vi "AD模拟量输入.vi"() -> ()   [LabVIEW 2010]
panel:
  in  "btn_反选":bool
  in  "btn_全选":bool
  in  "AD_16_5":sgl format="%.2f"
  in  "AD_16_4":sgl format="%.2f"
  in  "AD_16_3":sgl format="%.2f"
  in  "AD_16_2":sgl format="%.2f"
  in  "AD_16_1":sgl format="%.2f"
  in  "AD_15_5":sgl format="%.2f"
  in  "AD_15_4":sgl format="%.2f"
  in  "AD_15_3":sgl format="%.2f"
  in  "AD_15_2":sgl format="%.2f"
  in  "单选_AD_16":bool
  in  "单选_AD_15":bool
  in  "AD_15_1":sgl format="%.2f"
  in  "AD_14_5":sgl format="%.2f"
  in  "AD_14_4":sgl format="%.2f"
  in  "AD_14_3":sgl format="%.2f"
  in  "AD_14_2":sgl format="%.2f"
  in  "AD_14_1":sgl format="%.2f"
  in  "AD_13_5":sgl format="%.2f"
  in  "AD_13_4":sgl format="%.2f"
  in  "AD_13_3":sgl format="%.2f"
  in  "AD_13_2":sgl format="%.2f"
  in  "单选_AD_14":bool
  in  "单选_AD_13":bool
  in  "AD_13_1":sgl format="%.2f"
  in  "AD_12_5":sgl format="%.2f"
  in  "AD_12_4":sgl format="%.2f"
  in  "AD_12_3":sgl format="%.2f"
  in  "AD_12_2":sgl format="%.2f"
  in  "AD_12_1":sgl format="%.2f"
  in  "AD_11_5":sgl format="%.2f"
  in  "AD_11_4":sgl format="%.2f"
  in  "AD_11_3":sgl format="%.2f"
  in  "AD_11_2":sgl format="%.2f"
  in  "单选_AD_12":bool
  in  "单选_AD_11":bool
  in  "AD_11_1":sgl format="%.2f"
  in  "AD_10_5":sgl format="%.2f"
  in  "AD_10_4":sgl format="%.2f"
  in  "AD_10_3":sgl format="%.2f"
  in  "AD_10_2":sgl format="%.2f"
  in  "AD_10_1":sgl format="%.2f"
  in  "AD_9_5":sgl format="%.2f"
  in  "AD_9_4":sgl format="%.2f"
  in  "AD_9_3":sgl format="%.2f"
  in  "AD_9_2":sgl format="%.2f"
  in  "单选_AD_10":bool
  in  "单选_AD_9":bool
  in  "AD_9_1":sgl format="%.2f"
  in  "AD_8_5":sgl format="%.2f"
  in  "AD_8_4":sgl format="%.2f"
  in  "AD_8_3":sgl format="%.2f"
  in  "AD_8_2":sgl format="%.2f"
  in  "AD_8_1":sgl format="%.2f"
  in  "AD_7_5":sgl format="%.2f"
  in  "AD_7_4":sgl format="%.2f"
  in  "AD_7_3":sgl format="%.2f"
  in  "AD_7_2":sgl format="%.2f"
  in  "单选_AD_8":bool
  in  "单选_AD_7":bool
  in  "AD_7_1":sgl format="%.2f"
  in  "AD_6_5":sgl format="%.2f"
  in  "AD_6_4":sgl format="%.2f"
  in  "AD_6_3":sgl format="%.2f"
  in  "AD_6_2":sgl format="%.2f"
  in  "AD_6_1":sgl format="%.2f"
  in  "AD_5_5":sgl format="%.2f"
  in  "AD_5_4":sgl format="%.2f"
  in  "AD_5_3":sgl format="%.2f"
  in  "AD_5_2":sgl format="%.2f"
  in  "单选_AD_6":bool
  in  "单选_AD_5":bool
  in  "AD_5_1":sgl format="%.2f"
  in  "AD_4_5":sgl format="%.2f"
  in  "AD_4_4":sgl format="%.2f"
  in  "AD_4_3":sgl format="%.2f"
  in  "AD_4_2":sgl format="%.2f"
  in  "AD_4_1":sgl format="%.2f"
  in  "AD_3_5":sgl format="%.2f"
  in  "AD_3_4":sgl format="%.2f"
  in  "AD_3_3":sgl format="%.2f"
  in  "AD_3_2":sgl format="%.2f"
  in  "单选_AD_4":bool
  in  "单选_AD_3":bool
  in  "AD_3_1":sgl format="%.2f"
  in  "AD_2_5":sgl format="%.2f"
  in  "AD_2_4":sgl format="%.2f"
  in  "AD_2_3":sgl format="%.2f"
  in  "AD_2_2":sgl format="%.2f"
  in  "AD_2_1":sgl format="%.2f"
  in  "AD_1_5":sgl format="%.2f"
  in  "AD_1_4":sgl format="%.2f"
  in  "AD_1_3":sgl format="%.2f"
  in  "AD_1_2":sgl format="%.2f"
  in  "单选_AD_2":bool
  in  "单选_AD_1":bool
  in  "AD_1_1":sgl format="%.2f"
  in  "btn_取消":bool
  in  "btn_开始测试":bool
  # "第1路"
  # "输入值："
  # "输入值："
  # "第2路"
  # "第3路"
  # "输入值："
  # "输入值："
  # "第4路"
  # "第5路"
  # "输入值："
  # "输入值："
  # "第6路"
  # "第7路"
  # "输入值："
  # "输入值："
  # "第8路"
  # "第9路"
  # "输入值："
  # "输入值："
  # "第10路"
  # "第11路"
  # "输入值："
  # "输入值："
  # "第12路"
  # "第13路"
  # "输入值："
  # "输入值："
  # "第14路"
  # "第15路"
  # "输入值："
  # "输入值："
  # "第16路"
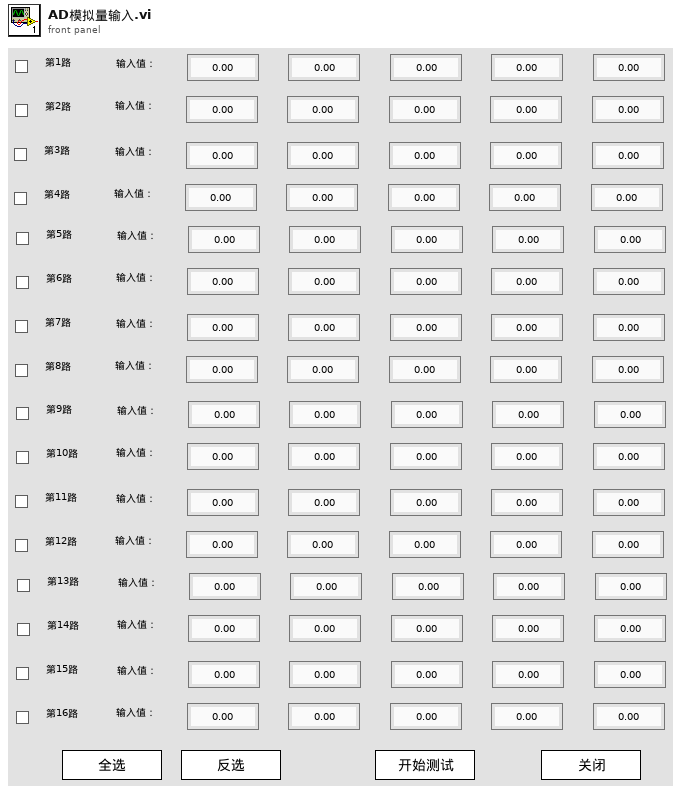
[diagram p1: front panel]
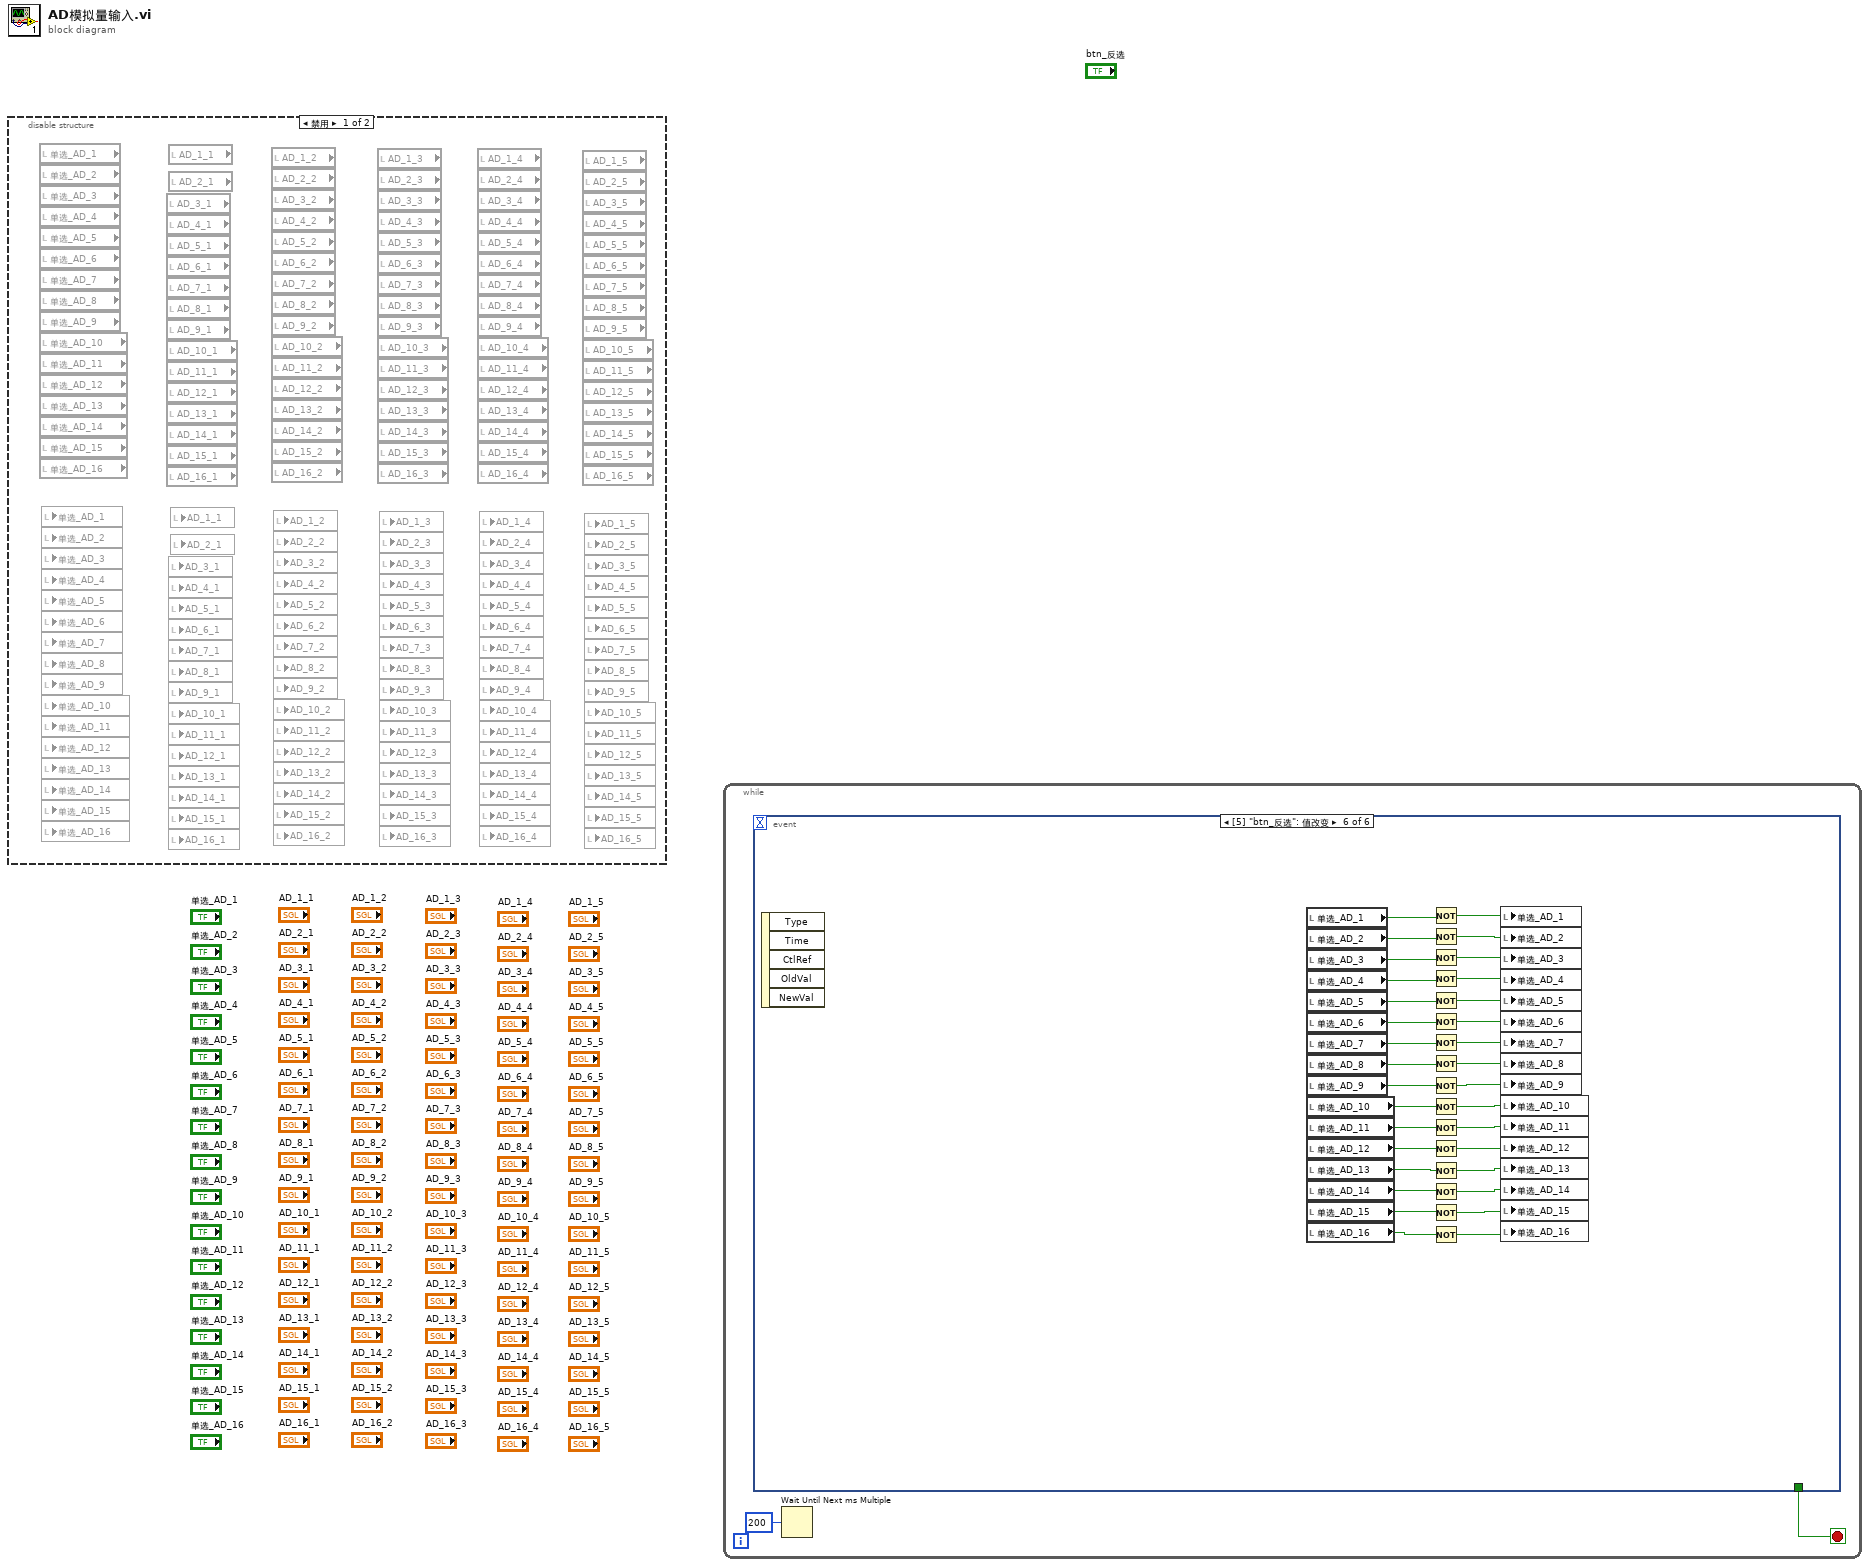
[diagram p0: block diagram]
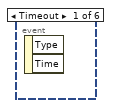
[diagram p3: hidden frame]
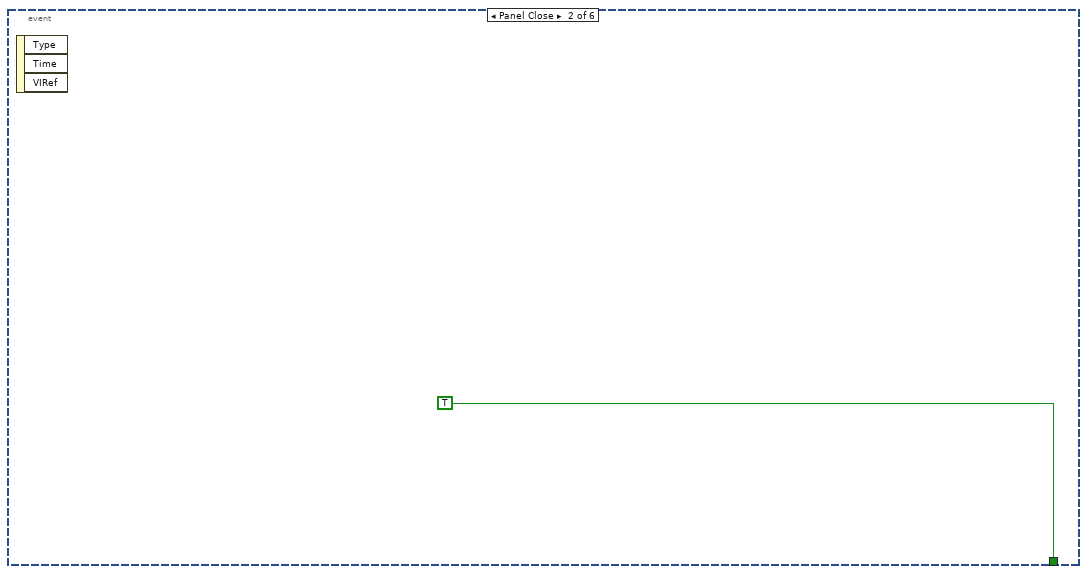
[diagram p4: hidden frame]
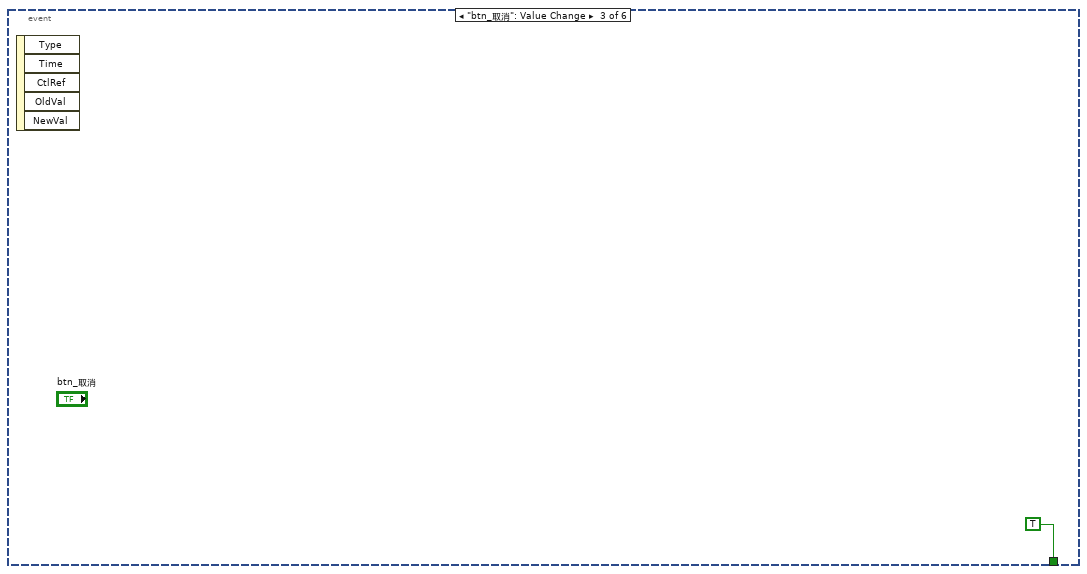
[diagram p5: hidden frame]
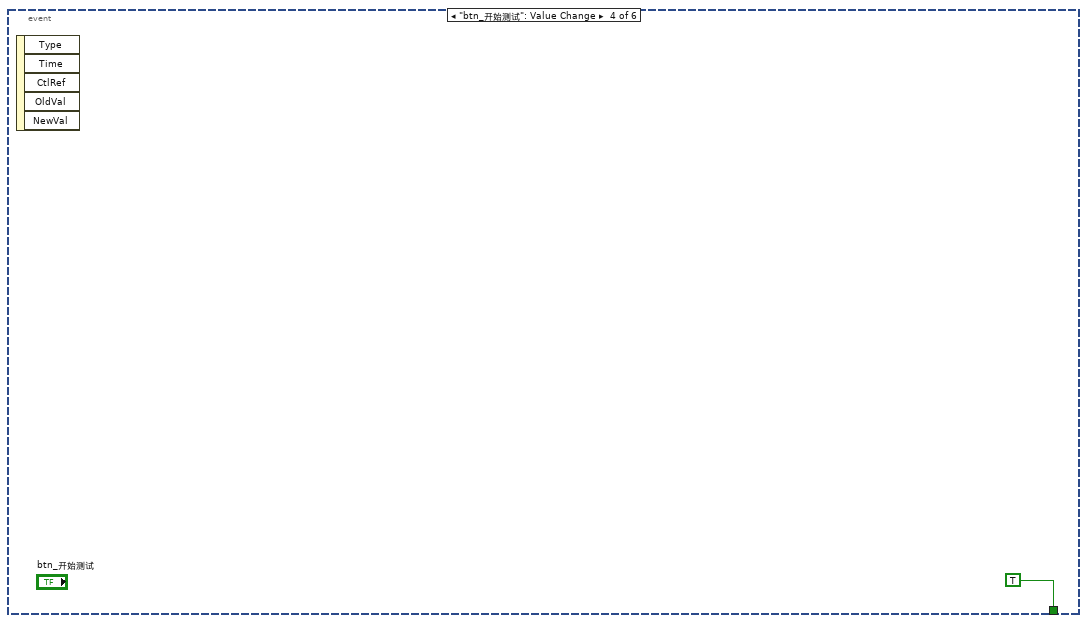
[diagram p6: hidden frame]
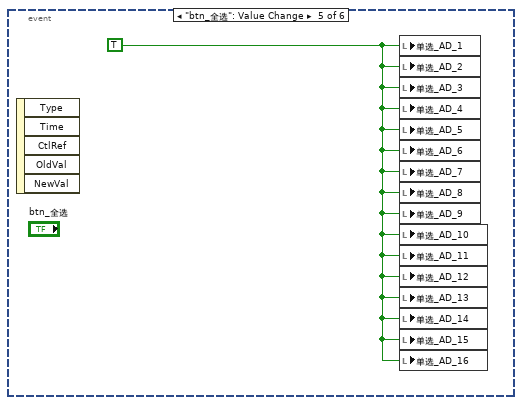
[diagram p7: hidden frame]
diagram:
  n1 = disable-structure shown="禁用" {
    frame Disabled {
      n2 = local read "单选_AD_1"() -> ()  [unwired: 1 out]
      n3 = local read "单选_AD_2"() -> ()  [unwired: 1 out]
      n4 = local read "单选_AD_3"() -> ()  [unwired: 1 out]
      n5 = local read "单选_AD_4"() -> ()  [unwired: 1 out]
      n6 = local read "单选_AD_5"() -> ()  [unwired: 1 out]
      n7 = local read "单选_AD_6"() -> ()  [unwired: 1 out]
      n8 = local read "单选_AD_7"() -> ()  [unwired: 1 out]
      n9 = local read "单选_AD_8"() -> ()  [unwired: 1 out]
      n10 = local read "单选_AD_9"() -> ()  [unwired: 1 out]
      n11 = local read "单选_AD_10"() -> ()  [unwired: 1 out]
      n12 = local read "单选_AD_11"() -> ()  [unwired: 1 out]
      n13 = local read "单选_AD_12"() -> ()  [unwired: 1 out]
      n14 = local read "单选_AD_13"() -> ()  [unwired: 1 out]
      n15 = local read "单选_AD_14"() -> ()  [unwired: 1 out]
      n16 = local read "单选_AD_15"() -> ()  [unwired: 1 out]
      n17 = local read "单选_AD_16"() -> ()  [unwired: 1 out]
      n18 = local read "单选_AD_1"() -> ()  [unwired: 1 in]
      n19 = local read "单选_AD_2"() -> ()  [unwired: 1 in]
      n20 = local read "单选_AD_3"() -> ()  [unwired: 1 in]
      n21 = local read "单选_AD_4"() -> ()  [unwired: 1 in]
      n22 = local read "单选_AD_5"() -> ()  [unwired: 1 in]
      n23 = local read "单选_AD_6"() -> ()  [unwired: 1 in]
      n24 = local read "单选_AD_7"() -> ()  [unwired: 1 in]
      n25 = local read "单选_AD_8"() -> ()  [unwired: 1 in]
      n26 = local read "单选_AD_9"() -> ()  [unwired: 1 in]
      n27 = local read "单选_AD_10"() -> ()  [unwired: 1 in]
      n28 = local read "单选_AD_11"() -> ()  [unwired: 1 in]
      n29 = local read "单选_AD_12"() -> ()  [unwired: 1 in]
      n30 = local read "单选_AD_13"() -> ()  [unwired: 1 in]
      n31 = local read "单选_AD_14"() -> ()  [unwired: 1 in]
      n32 = local read "单选_AD_15"() -> ()  [unwired: 1 in]
      n33 = local read "单选_AD_16"() -> ()  [unwired: 1 in]
      n34 = local read "AD_3_1"() -> ()  [unwired: 1 out]
      n35 = local read "AD_4_1"() -> ()  [unwired: 1 out]
      n36 = local read "AD_5_1"() -> ()  [unwired: 1 out]
      n37 = local read "AD_6_1"() -> ()  [unwired: 1 out]
      n38 = local read "AD_7_1"() -> ()  [unwired: 1 out]
      n39 = local read "AD_8_1"() -> ()  [unwired: 1 out]
      n40 = local read "AD_9_1"() -> ()  [unwired: 1 out]
      n41 = local read "AD_10_1"() -> ()  [unwired: 1 out]
      n42 = local read "AD_11_1"() -> ()  [unwired: 1 out]
      n43 = local read "AD_12_1"() -> ()  [unwired: 1 out]
      n44 = local read "AD_13_1"() -> ()  [unwired: 1 out]
      n45 = local read "AD_14_1"() -> ()  [unwired: 1 out]
      n46 = local read "AD_15_1"() -> ()  [unwired: 1 out]
      n47 = local read "AD_16_1"() -> ()  [unwired: 1 out]
      n48 = local read "AD_1_1"() -> ()  [unwired: 1 out]
      n49 = local read "AD_2_1"() -> ()  [unwired: 1 out]
      n50 = local read "AD_3_1"() -> ()  [unwired: 1 in]
      n51 = local read "AD_4_1"() -> ()  [unwired: 1 in]
      n52 = local read "AD_5_1"() -> ()  [unwired: 1 in]
      n53 = local read "AD_6_1"() -> ()  [unwired: 1 in]
      n54 = local read "AD_7_1"() -> ()  [unwired: 1 in]
      n55 = local read "AD_8_1"() -> ()  [unwired: 1 in]
      n56 = local read "AD_9_1"() -> ()  [unwired: 1 in]
      n57 = local read "AD_10_1"() -> ()  [unwired: 1 in]
      n58 = local read "AD_11_1"() -> ()  [unwired: 1 in]
      n59 = local read "AD_12_1"() -> ()  [unwired: 1 in]
      n60 = local read "AD_13_1"() -> ()  [unwired: 1 in]
      n61 = local read "AD_14_1"() -> ()  [unwired: 1 in]
      n62 = local read "AD_15_1"() -> ()  [unwired: 1 in]
      n63 = local read "AD_16_1"() -> ()  [unwired: 1 in]
      n64 = local read "AD_1_1"() -> ()  [unwired: 1 in]
      n65 = local read "AD_2_1"() -> ()  [unwired: 1 in]
      n66 = local read "AD_1_2"() -> ()  [unwired: 1 out]
      n67 = local read "AD_2_2"() -> ()  [unwired: 1 out]
      n68 = local read "AD_3_2"() -> ()  [unwired: 1 out]
      n69 = local read "AD_4_2"() -> ()  [unwired: 1 out]
      n70 = local read "AD_5_2"() -> ()  [unwired: 1 out]
      n71 = local read "AD_6_2"() -> ()  [unwired: 1 out]
      n72 = local read "AD_7_2"() -> ()  [unwired: 1 out]
      n73 = local read "AD_8_2"() -> ()  [unwired: 1 out]
      n74 = local read "AD_9_2"() -> ()  [unwired: 1 out]
      n75 = local read "AD_10_2"() -> ()  [unwired: 1 out]
      n76 = local read "AD_11_2"() -> ()  [unwired: 1 out]
      n77 = local read "AD_12_2"() -> ()  [unwired: 1 out]
      n78 = local read "AD_13_2"() -> ()  [unwired: 1 out]
      n79 = local read "AD_14_2"() -> ()  [unwired: 1 out]
      n80 = local read "AD_15_2"() -> ()  [unwired: 1 out]
      n81 = local read "AD_16_2"() -> ()  [unwired: 1 out]
      n82 = local read "AD_1_2"() -> ()  [unwired: 1 in]
      n83 = local read "AD_2_2"() -> ()  [unwired: 1 in]
      n84 = local read "AD_3_2"() -> ()  [unwired: 1 in]
      n85 = local read "AD_4_2"() -> ()  [unwired: 1 in]
      n86 = local read "AD_5_2"() -> ()  [unwired: 1 in]
      n87 = local read "AD_6_2"() -> ()  [unwired: 1 in]
      n88 = local read "AD_7_2"() -> ()  [unwired: 1 in]
      n89 = local read "AD_8_2"() -> ()  [unwired: 1 in]
      n90 = local read "AD_9_2"() -> ()  [unwired: 1 in]
      n91 = local read "AD_10_2"() -> ()  [unwired: 1 in]
      n92 = local read "AD_11_2"() -> ()  [unwired: 1 in]
      n93 = local read "AD_12_2"() -> ()  [unwired: 1 in]
      n94 = local read "AD_13_2"() -> ()  [unwired: 1 in]
      n95 = local read "AD_14_2"() -> ()  [unwired: 1 in]
      n96 = local read "AD_15_2"() -> ()  [unwired: 1 in]
      n97 = local read "AD_16_2"() -> ()  [unwired: 1 in]
      n98 = local read "AD_1_3"() -> ()  [unwired: 1 out]
      n99 = local read "AD_2_3"() -> ()  [unwired: 1 out]
      n100 = local read "AD_3_3"() -> ()  [unwired: 1 out]
      n101 = local read "AD_4_3"() -> ()  [unwired: 1 out]
      n102 = local read "AD_5_3"() -> ()  [unwired: 1 out]
      n103 = local read "AD_6_3"() -> ()  [unwired: 1 out]
      n104 = local read "AD_7_3"() -> ()  [unwired: 1 out]
      n105 = local read "AD_8_3"() -> ()  [unwired: 1 out]
      n106 = local read "AD_9_3"() -> ()  [unwired: 1 out]
      n107 = local read "AD_10_3"() -> ()  [unwired: 1 out]
      n108 = local read "AD_11_3"() -> ()  [unwired: 1 out]
      n109 = local read "AD_12_3"() -> ()  [unwired: 1 out]
      n110 = local read "AD_13_3"() -> ()  [unwired: 1 out]
      n111 = local read "AD_14_3"() -> ()  [unwired: 1 out]
      n112 = local read "AD_15_3"() -> ()  [unwired: 1 out]
      n113 = local read "AD_16_3"() -> ()  [unwired: 1 out]
      n114 = local read "AD_1_3"() -> ()  [unwired: 1 in]
      n115 = local read "AD_2_3"() -> ()  [unwired: 1 in]
      n116 = local read "AD_3_3"() -> ()  [unwired: 1 in]
      n117 = local read "AD_4_3"() -> ()  [unwired: 1 in]
      n118 = local read "AD_5_3"() -> ()  [unwired: 1 in]
      n119 = local read "AD_6_3"() -> ()  [unwired: 1 in]
      n120 = local read "AD_7_3"() -> ()  [unwired: 1 in]
      n121 = local read "AD_8_3"() -> ()  [unwired: 1 in]
      n122 = local read "AD_9_3"() -> ()  [unwired: 1 in]
      n123 = local read "AD_10_3"() -> ()  [unwired: 1 in]
      n124 = local read "AD_11_3"() -> ()  [unwired: 1 in]
      n125 = local read "AD_12_3"() -> ()  [unwired: 1 in]
      n126 = local read "AD_13_3"() -> ()  [unwired: 1 in]
      n127 = local read "AD_14_3"() -> ()  [unwired: 1 in]
      n128 = local read "AD_15_3"() -> ()  [unwired: 1 in]
      n129 = local read "AD_16_3"() -> ()  [unwired: 1 in]
      n130 = local read "AD_1_4"() -> ()  [unwired: 1 out]
      n131 = local read "AD_2_4"() -> ()  [unwired: 1 out]
      n132 = local read "AD_3_4"() -> ()  [unwired: 1 out]
      n133 = local read "AD_4_4"() -> ()  [unwired: 1 out]
      n134 = local read "AD_5_4"() -> ()  [unwired: 1 out]
      n135 = local read "AD_6_4"() -> ()  [unwired: 1 out]
      n136 = local read "AD_7_4"() -> ()  [unwired: 1 out]
      n137 = local read "AD_8_4"() -> ()  [unwired: 1 out]
      n138 = local read "AD_9_4"() -> ()  [unwired: 1 out]
      n139 = local read "AD_10_4"() -> ()  [unwired: 1 out]
      n140 = local read "AD_11_4"() -> ()  [unwired: 1 out]
      n141 = local read "AD_12_4"() -> ()  [unwired: 1 out]
      n142 = local read "AD_13_4"() -> ()  [unwired: 1 out]
      n143 = local read "AD_14_4"() -> ()  [unwired: 1 out]
      n144 = local read "AD_15_4"() -> ()  [unwired: 1 out]
      n145 = local read "AD_16_4"() -> ()  [unwired: 1 out]
      n146 = local read "AD_1_4"() -> ()  [unwired: 1 in]
      n147 = local read "AD_2_4"() -> ()  [unwired: 1 in]
      n148 = local read "AD_3_4"() -> ()  [unwired: 1 in]
      n149 = local read "AD_4_4"() -> ()  [unwired: 1 in]
      n150 = local read "AD_5_4"() -> ()  [unwired: 1 in]
      n151 = local read "AD_6_4"() -> ()  [unwired: 1 in]
      n152 = local read "AD_7_4"() -> ()  [unwired: 1 in]
      n153 = local read "AD_8_4"() -> ()  [unwired: 1 in]
      n154 = local read "AD_9_4"() -> ()  [unwired: 1 in]
      n155 = local read "AD_10_4"() -> ()  [unwired: 1 in]
      n156 = local read "AD_11_4"() -> ()  [unwired: 1 in]
      n157 = local read "AD_12_4"() -> ()  [unwired: 1 in]
      n158 = local read "AD_13_4"() -> ()  [unwired: 1 in]
      n159 = local read "AD_14_4"() -> ()  [unwired: 1 in]
      n160 = local read "AD_15_4"() -> ()  [unwired: 1 in]
      n161 = local read "AD_16_4"() -> ()  [unwired: 1 in]
      n162 = local read "AD_1_5"() -> ()  [unwired: 1 out]
      n163 = local read "AD_2_5"() -> ()  [unwired: 1 out]
      n164 = local read "AD_3_5"() -> ()  [unwired: 1 out]
      n165 = local read "AD_4_5"() -> ()  [unwired: 1 out]
      n166 = local read "AD_5_5"() -> ()  [unwired: 1 out]
      n167 = local read "AD_6_5"() -> ()  [unwired: 1 out]
      n168 = local read "AD_7_5"() -> ()  [unwired: 1 out]
      n169 = local read "AD_8_5"() -> ()  [unwired: 1 out]
      n170 = local read "AD_9_5"() -> ()  [unwired: 1 out]
      n171 = local read "AD_10_5"() -> ()  [unwired: 1 out]
      n172 = local read "AD_11_5"() -> ()  [unwired: 1 out]
      n173 = local read "AD_12_5"() -> ()  [unwired: 1 out]
      n174 = local read "AD_13_5"() -> ()  [unwired: 1 out]
      n175 = local read "AD_14_5"() -> ()  [unwired: 1 out]
      n176 = local read "AD_15_5"() -> ()  [unwired: 1 out]
      n177 = local read "AD_16_5"() -> ()  [unwired: 1 out]
      n178 = local read "AD_1_5"() -> ()  [unwired: 1 in]
      n179 = local read "AD_2_5"() -> ()  [unwired: 1 in]
      n180 = local read "AD_3_5"() -> ()  [unwired: 1 in]
      n181 = local read "AD_4_5"() -> ()  [unwired: 1 in]
      n182 = local read "AD_5_5"() -> ()  [unwired: 1 in]
      n183 = local read "AD_6_5"() -> ()  [unwired: 1 in]
      n184 = local read "AD_7_5"() -> ()  [unwired: 1 in]
      n185 = local read "AD_8_5"() -> ()  [unwired: 1 in]
      n186 = local read "AD_9_5"() -> ()  [unwired: 1 in]
      n187 = local read "AD_10_5"() -> ()  [unwired: 1 in]
      n188 = local read "AD_11_5"() -> ()  [unwired: 1 in]
      n189 = local read "AD_12_5"() -> ()  [unwired: 1 in]
      n190 = local read "AD_13_5"() -> ()  [unwired: 1 in]
      n191 = local read "AD_14_5"() -> ()  [unwired: 1 in]
      n192 = local read "AD_15_5"() -> ()  [unwired: 1 in]
      n193 = local read "AD_16_5"() -> ()  [unwired: 1 in]
    }
    frame Enabled {
    }
  }
  n194 = while {
    stop <- w2 stop-if-true
    n195 = event shown="[5] \"btn_反选\": 值改变" {
      selector: _ -> [_ _ _ _ _ _]
      dyn-events: _ -> [_ _ _ _ _ _]
      timeout: _ -> [_ _ _ _ _ _]
      tunnel: [_ TRUE TRUE TRUE _ _] -> w2
      event Timeout {
        n196 = event-data() -> ()  [unwired: 1 in, 2 out]
      }
      event Panel Close {
        n197 = event-data() -> ()  [unwired: 1 in, 3 out]
      }
      event "btn_取消": Value Change {
        n198 = event-data() -> ()  [unwired: 1 in, 5 out]
      }
      event "btn_开始测试": Value Change {
        n199 = event-data() -> ()  [unwired: 1 in, 5 out]
      }
      event "btn_全选": Value Change {
        w6 = TRUE ("单选_AD_1")
        n200 = event-data() -> ()  [unwired: 1 in, 5 out]
        n201 = local write "单选_AD_1"(w6) -> ()
        n202 = local write "单选_AD_2"(w6) -> ()
        n203 = local write "单选_AD_3"(w6) -> ()
        n204 = local write "单选_AD_4"(w6) -> ()
        n205 = local write "单选_AD_5"(w6) -> ()
        n206 = local write "单选_AD_6"(w6) -> ()
        n207 = local write "单选_AD_7"(w6) -> ()
        n208 = local write "单选_AD_8"(w6) -> ()
        n209 = local write "单选_AD_9"(w6) -> ()
        n210 = local write "单选_AD_10"(w6) -> ()
        n211 = local write "单选_AD_11"(w6) -> ()
        n212 = local write "单选_AD_12"(w6) -> ()
        n213 = local write "单选_AD_13"(w6) -> ()
        n214 = local write "单选_AD_14"(w6) -> ()
        n215 = local write "单选_AD_15"(w6) -> ()
        n216 = local write "单选_AD_16"(w6) -> ()
      }
      event "btn_反选": Value Change {
        n217 = event-data() -> ()  [unwired: 1 in, 5 out]
        n218 = local read "单选_AD_1"() -> (w38:bool)
        n219 = local read "单选_AD_2"() -> (w37:bool)
        n220 = local read "单选_AD_3"() -> (w36:bool)
        n221 = local read "单选_AD_4"() -> (w35:bool)
        n222 = local read "单选_AD_5"() -> (w34:bool)
        n223 = local read "单选_AD_6"() -> (w33:bool)
        n224 = local read "单选_AD_7"() -> (w32:bool)
        n225 = local read "单选_AD_8"() -> (w31:bool)
        n226 = local read "单选_AD_9"() -> (w30:bool)
        n227 = local read "单选_AD_10"() -> (w29:bool)
        n228 = local read "单选_AD_11"() -> (w28:bool)
        n229 = local read "单选_AD_12"() -> (w27:bool)
        n230 = local read "单选_AD_13"() -> (w26:bool)
        n231 = local read "单选_AD_14"() -> (w25:bool)
        n232 = local read "单选_AD_15"() -> (w24:bool)
        n233 = local read "单选_AD_16"() -> (w23:bool)
        n234 = Not(x=w38) -> (.not. x?=w22:bool)
        n235 = Not(x=w37) -> (.not. x?=w21:bool)
        n236 = Not(x=w36) -> (.not. x?=w20:bool)
        n237 = Not(x=w35) -> (.not. x?=w19:bool)
        n238 = Not(x=w34) -> (.not. x?=w18:bool)
        n239 = Not(x=w33) -> (.not. x?=w17:bool)
        n240 = Not(x=w32) -> (.not. x?=w16:bool)
        n241 = Not(x=w31) -> (.not. x?=w15:bool)
        n242 = Not(x=w30) -> (.not. x?=w14:bool)
        n243 = Not(x=w29) -> (.not. x?=w13:bool)
        n244 = Not(x=w28) -> (.not. x?=w12:bool)
        n245 = Not(x=w27) -> (.not. x?=w11:bool)
        n246 = Not(x=w26) -> (.not. x?=w10:bool)
        n247 = Not(x=w25) -> (.not. x?=w9:bool)
        n248 = Not(x=w24) -> (.not. x?=w8:bool)
        n249 = Not(x=w23) -> (.not. x?=w7:bool)
        n250 = local write "单选_AD_1"(w22) -> ()
        n251 = local write "单选_AD_2"(w21) -> ()
        n252 = local write "单选_AD_3"(w20) -> ()
        n253 = local write "单选_AD_4"(w19) -> ()
        n254 = local write "单选_AD_5"(w18) -> ()
        n255 = local write "单选_AD_6"(w17) -> ()
        n256 = local write "单选_AD_7"(w16) -> ()
        n257 = local write "单选_AD_8"(w15) -> ()
        n258 = local write "单选_AD_9"(w14) -> ()
        n259 = local write "单选_AD_10"(w13) -> ()
        n260 = local write "单选_AD_11"(w12) -> ()
        n261 = local write "单选_AD_12"(w11) -> ()
        n262 = local write "单选_AD_13"(w10) -> ()
        n263 = local write "单选_AD_14"(w9) -> ()
        n264 = local write "单选_AD_15"(w8) -> ()
        n265 = local write "单选_AD_16"(w7) -> ()
      }
    }
    n266 = Wait Until Next ms Multiple(millisecond multiple=u32 200 ("毫秒倍数")) -> ()  [unwired: 1 out]
  }
